vi "navX Example (SPI - I2C).vi"() -> ()   [LabVIEW 2014]
uses:
  navX-MXP Library/COMMON/TypeDefs/Value TypeDefs/navX Update Rate.ctl
  navX-MXP Library/COMMON/TypeDefs/Data TypeDefs/navX Vector Data.ctl
  navX-MXP Library/COMMON/TypeDefs/Data TypeDefs/navX YPRH Data.ctl
  navX-MXP Library/COMMON/TypeDefs/Data TypeDefs/navX Quaternion Data.ctl
  navX-MXP Library/COMMON/TypeDefs/Data TypeDefs/navX Status Data.ctl
  navX-MXP Library/COMMON/TypeDefs/Value TypeDefs/navX NAVX_OP_STATUS.ctl
  navX-MXP Library/COMMON/TypeDefs/Value TypeDefs/navX NAVX_CAL_STATUS.ctl
  navX-MXP Library/COMMON/TypeDefs/Value TypeDefs/navX NAVX_SENSOR_STATUS.ctl
  navX-MXP Library/COMMON/TypeDefs/Value TypeDefs/navX Interface Protocol.ctl
  <vilib>/Platform/TimedLoop/XDataNode/timing_clust.ctl
  <vilib>/Platform/TimedLoop/XDataNode/nitl_modes.ctl
  <vilib>/Platform/TimedLoop/XDataNode/wakeup.ctl
  <vilib>/platform/TimedLoop/XDataNode/XDataNode.xnode
  navX-MXP Library/navX-MXP IMU.lvlib
  <vilib>/Platform/TimedLoop/XDataNode/XDNodeRunTimeDep.lvlib
panel:
  out "Timestamp":u32
  out "Fused Heading":dbl(knob) scale=0.0..360.0
  out "MPU Temperature (Centigrade)":dbl(slide) scale=20.0..40.0
  in  "navX Interface Protocol":T1
  out "Status":T2={"Update Rate Hz"=0, "Accelerometer Full-Scale Range"=0, "Gyro Full-Scale Range"=0, "NAVX_OP_STATUS"=0, "NAVX_CAL_STATUS"=0, "NAVX_SELFTEST_STATUS"=80, "NAVX_SENSOR_STATUS"={"MOVING"=FALSE, "YAW_STABLE"=FALSE, "MAG_DISTURBANCE"=FALSE, "ALTITUDE_VALID"=FALSE, "SEALEVEL_PRESS_SET"=FALSE, "FUSED_HEADING_VALID"=FALSE}} {"NAVX_OP_STATUS" items=["INITIALIZING", "SELFTEST_IN_PROGRESS", "ERROR", "IMU_AUTOCAL_IN_PROGRESS", "NORMAL"]; "NAVX_CAL_STATUS" items=["IMU_CAL_STATE_MASK"=3, "IMU_CAL_INPROGRESS"=0, "IMU_CAL_ACCUMULATE"=1, "IMU_CAL_COMPLETE"=2, "MAG_CAL_COMPLETE"=4, "BARO_CAL_COMPLETE"=8]}
  out "RawMag":T6
  out "RawGyro":T6
  out "RawAccel":T6
  out "Quaternion":T7
  out "YPRH":T8
  out "Acceleration":T6
  out "Valid?":bool
  in  "stop":bool
  out "Opened":bool
  in  "Update Rate (4Hz-60Hz)":T9=40 min=4 max=50 step=1
  # "SPI/I2C"
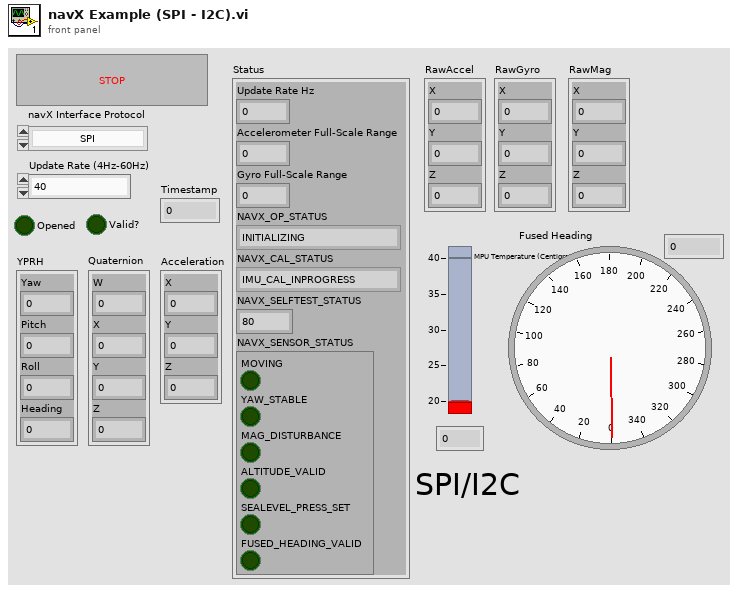
[diagram p1: front panel]
types:
  T1 = typedef "navX-MXP IMU.lvlib/navX Interface Protocol.ctl" = enum16{"SPI", "I2C"}
  T2 = typedef "navX-MXP IMU.lvlib/navX Status Data.ctl" = cluster{"Update Rate Hz":u8, "Accelerometer Full-Scale Range":u8, "Gyro Full-Scale Range":u16, "NAVX_OP_STATUS":T3, "NAVX_CAL_STATUS":T4, "NAVX_SELFTEST_STATUS":u8, "NAVX_SENSOR_STATUS":T5}
  T3 = typedef "navX-MXP IMU.lvlib/navX NAVX_OP_STATUS.ctl" = u8
  T4 = typedef "navX-MXP IMU.lvlib/navX NAVX_CAL_STATUS.ctl" = u8
  T5 = typedef "navX-MXP IMU.lvlib/navX NAVX_SENSOR_STATUS.ctl" = cluster{"MOVING":bool, "YAW_STABLE":bool, "MAG_DISTURBANCE":bool, "ALTITUDE_VALID":bool, "SEALEVEL_PRESS_SET":bool, "FUSED_HEADING_VALID":bool}
  T6 = typedef "navX-MXP IMU.lvlib/navX Vector Data.ctl" = cluster{"X":dbl, "Y":dbl, "Z":dbl}
  T7 = typedef "navX-MXP IMU.lvlib/navX Quaternion Data.ctl" = cluster{"W":dbl, "X":dbl, "Y":dbl, "Z":dbl}
  T8 = typedef "navX-MXP IMU.lvlib/navX YPRH Data.ctl" = cluster{"Yaw":dbl, "Pitch":dbl, "Roll":dbl, "Heading":dbl}
  T9 = typedef "navX-MXP IMU.lvlib/navX Update Rate.ctl" = u8
  T10 = typedef "navX-MXP IMU.lvlib/navX Device TypeDef.ctl" = cluster{"navX Interface Protocol":T1, "navX Interface Protocol TypeDefs":cluster{"SPIDevRef":T11, "I2CDevRef":T14}, "navX System Information":cluster{"Board Information":T16, "Status":T2, "Offsets":T17}, "navX Common Information":cluster{"Update Rate (4Hz-60Hz)":T9, "refnum name":string, "error":errorcluster}}
  T11 = typedef "WPI_SPIDevRef.ctl" = cluster{"DevStatus":errorcluster, "Handle":i32, "Controller":T12, "SPI Bus":T13}
  T12 = typedef "FPGA_TypedefDigitalModule.ctl" = enum16{"Controller 1"}
  T13 = typedef "spi_bus.ctl" = enum16{"SPI On-Board, CS0", "SPI On-Board, CS1", "SPI On-Board, CS2", "SPI On-Board, CS3", "SPI MXP", "Invalid"}
  T14 = typedef "WPI_I2CDevRef.ctl" = cluster{"DevStatus":errorcluster, "Controller":T12, "Device Address":u8, "Handle":i32, "I2C Bus":T15}
  T15 = typedef "i2c_bus.ctl" = enum16{"I2C On-Board", "I2C MXP", "Invalid"}
  T16 = typedef "navX-MXP IMU.lvlib/navX Board Information.ctl" = cluster{"WhoAmI (50 | 0x32)":u8, "Board Revision":u8, "Firmware Major Version":u8, "Firmware Minor Version":u8}
  T17 = typedef "navX-MXP IMU.lvlib/navX Offsets Data.ctl" = cluster{"Yaw":dbl, "Quat W":dbl, "Quat X":dbl, "Quat Y":dbl, "Quat Z":dbl}
  T18 = typedef "XDNodeRunTimeDep.lvlib/timing_clust.ctl" = cluster{"Expected End [f-1]":u64, "Actual End [f-1]":u64, "Finished Late? [f-1]":bool, "Expected End [i-1]":u64, "Actual End [i-1]":u64, "Finished Late? [i-1]":bool, "Expected Start [i]":u64, "Actual Start [i]":u64, "Expected Start [f]":u64, "Actual Start [f]":u64, "Source Name":string, "Structure Name":string, "Period":i64, "Deadline":i64, "Offset":i64, "Start":i64, "Priority":i32, "Timeout":i32, "Mode":T19, "Wakeup Reason":T20, "Error":errorcluster, "Source Type":string, "Secondary Source Type":string, "Global End Time":u64, "Global Start Time":u64, "Frame Duration":u64, "Iteration Duration":u64, "Assigned CPU":i32, "I/O Scan Engine Mode":u32}
  T19 = typedef "XDNodeRunTimeDep.lvlib/nitl_modes.ctl" = enum32{"No Change", "Process missed periods, maintain original phase", "Discard missed periods, maintain original phase", "Process missed periods, ignore original phase", "Discard missed periods, ignore original phase"}
  T20 = typedef "XDNodeRunTimeDep.lvlib/wakeup.ctl" = enum32{"Normal", "Aborted", "Asynchronous wakeup", "Timing source error", "Timed loop error", "Timeout"}
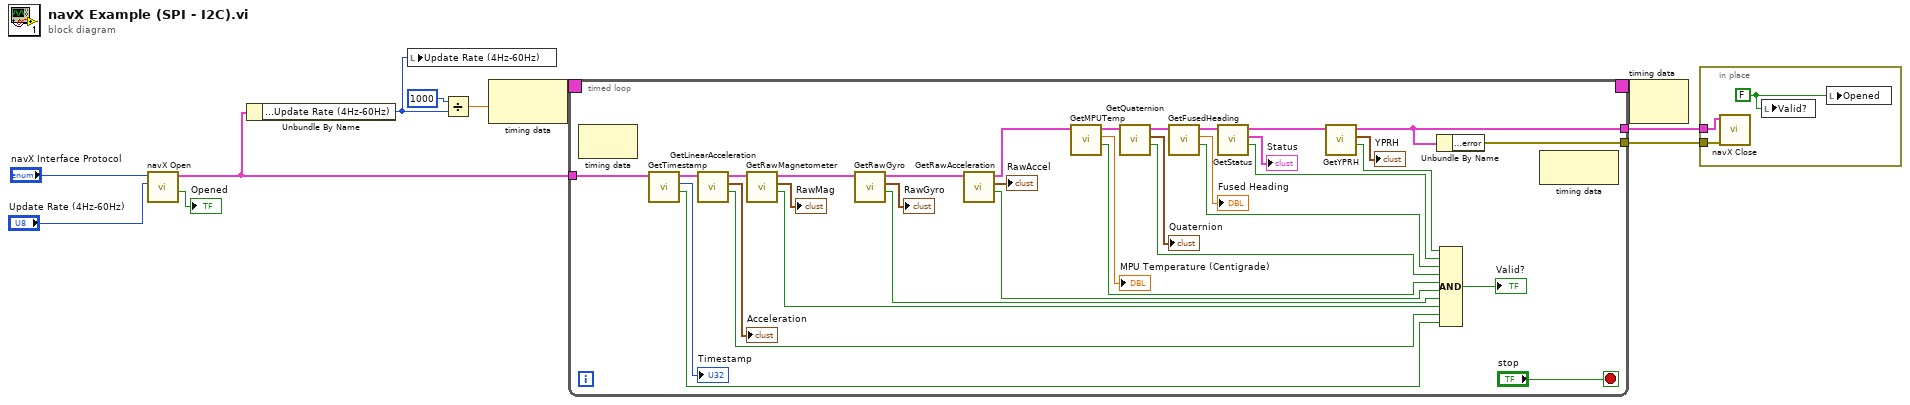
[diagram p0: block diagram]
diagram:
  n1 = call "navX Open.vi"("Update Rate (4Hz-60Hz)"="Update Rate (4Hz-60Hz)", "navX Interface Protocol"="navX Interface Protocol") -> ("Opened?"=→"Opened":bool, "navX Device TypeDef"=w3:T10)  [unwired: 7 in, 1 out]
  n2 = Unbundle By Name(w3) -> ("navX Common Information.Update Rate (4Hz-60Hz)"=w7:T9)
  n3 = local write "Update Rate (4Hz-60Hz)"(w7) -> ()
  n4 = Divide(x=1000, y=w7) -> (x/y=w4:dbl)
  n5 = node-c288(w4) -> (w6:T18)
  n6 = timed-loop {
    timing: w6 -> [_]
    timing-out: [_] -> w5
    tunnel: w3 -> [w40]
    tunnel: [w42] -> w2
    tunnel: [w41] -> w1
    stop <- "stop" stop-if-true
    n7 = node-c288() -> ()  [unwired: 1 in, 1 out]
    n8 = call "GetTimestamp.vi"("navX Device TypeDef"=w40) -> ("Valid?"=w12:bool, "Timestamp"=→"Timestamp":u32, "navX Device TypeDef"=w14:T10)  [unwired: 8 in]
    n9 = call "GetLinearAcceleration.vi"("navX Device TypeDef"=w14) -> ("Valid?"=w16:bool, "Linear Acceleration"=→"Acceleration":T6, "navX Device TypeDef"=w18:T10)  [unwired: 8 in]
    n10 = call "GetRawMagnetometer.vi"("navX Device TypeDef"=w18) -> ("Valid?"=w19:bool, "Raw Magnetometer"=→"RawMag":T6, "navX Device TypeDef"=w21:T10)  [unwired: 8 in]
    n11 = call "GetRawGyro.vi"("navX Device TypeDef"=w21) -> ("Valid?"=w22:bool, "Raw Gyro"=→"RawGyro":T6, "navX Device TypeDef"=w24:T10)  [unwired: 8 in]
    n12 = call "GetRawAcceleration.vi"("navX Device TypeDef"=w24) -> ("Valid?"=w25:bool, "Raw Acceleration"=→"RawAccel":T6, "navX Device TypeDef"=w27:T10)  [unwired: 8 in]
    n13 = call "GetMPUTemp.vi"("navX Device TypeDef"=w27) -> ("Valid?"=w28:bool, "MPU Temperature (Centigrade)"=→"MPU Temperature (Centigrade)":dbl, "navX Device TypeDef"=w30:T10)  [unwired: 8 in]
    n14 = call "GetQuaternion.vi"("navX Device TypeDef"=w30) -> ("Valid?"=w32:bool, "Quaternion"=→"Quaternion":T7, "navX Device TypeDef"=w33:T10)  [unwired: 8 in]
    n15 = call "GetFusedHeading.vi"("navX Device TypeDef"=w33) -> ("Valid?"=w34:bool, "Fused Heading"=→"Fused Heading":dbl, "navX Device TypeDef"=w35:T10)  [unwired: 8 in]
    n16 = call "GetStatus.vi"("navX Device TypeDef"=w35) -> ("Valid?"=w36:bool, "Status"=→"Status":T2, "navX Device TypeDef"=w39:T10)  [unwired: 8 in]
    n17 = call "GetYPRH.vi"("navX Device TypeDef"=w39) -> ("Valid?"=w44:bool, "YPRH"=→"YPRH":T8, "navX Device TypeDef"=w42:T10)  [unwired: 8 in]
    n18 = Unbundle By Name(w42) -> ("navX Common Information.error"=w41:errorcluster)
    n19 = Compound Arithmetic op=AND(w44, w36, w34, w32, w28, w25, w22, w19, w16, w12) -> (→"Valid?":bool)
    n20 = node-c288() -> ()  [unwired: 1 in, 1 out]
  }
  n21 = node-c288(w5) -> ()  [unwired: 1 out]
  n22 = in-place {
    in-place-border: w2 -> [w50]
    in-place-border: w1 -> [w49]
    w48 = FALSE ("Valid?")
    n23 = call "navX Close.vi"("error in (no error)"=w49, "navX Device TypeDef"=w50) -> ()  [unwired: 9 in, 1 out]
    n24 = local write "Valid?"(w48) -> ()
    n25 = local write "Opened"(w48) -> ()
  }
